vi "Initialize Sessions - 1Sess.vi"(6 "initialize and close session behavior":T2, 7 "visa open timeout":u32, 8 "error in":errorcluster, 9 "access mode":T1 items=["VISA Defaults"=0, "Exclusive Lock"=1, "Load Configured Settings"=4], 10 "instrument type id":string, 11 "session reservation in":refnum<class "Session Reservation.lvclass">) -> (0 "error out":errorcluster, 1 "channel list":string, 2 "session":refnum<visa-resource-name>, 3 "session reservation out":refnum<class "Session Reservation.lvclass">)   [LabVIEW 2020, in "NI Session Management VISA.lvlib"]
doc: "Create a VISA session from the <b>session reservation in</b> and the <b>instrument type id</b>. The <b>instrument type id</b> must match the Instrument Type Id for the custom VISA instrument in the pin map. Returns an error if more than one VISA session has been reserved. Use \"Create Sesssion - NSess.vi\" for multiple sessions."
uses:
  NI Session Management VISA.lvlib
  7f77feb2-d2b5-4acd-8f0f-f1b24b7d1641.vi
  Session Factory/Session Factory.lvclass
  Clients/Session Management V1/Session Reservation/Session Reservation.lvclass
  Clients/Session Management V1/Session Reservation/Initialize and Close Session Behavior.ctl
  <vilib>/Instr/_visa.llb/VISA Open Access Mode.ctl
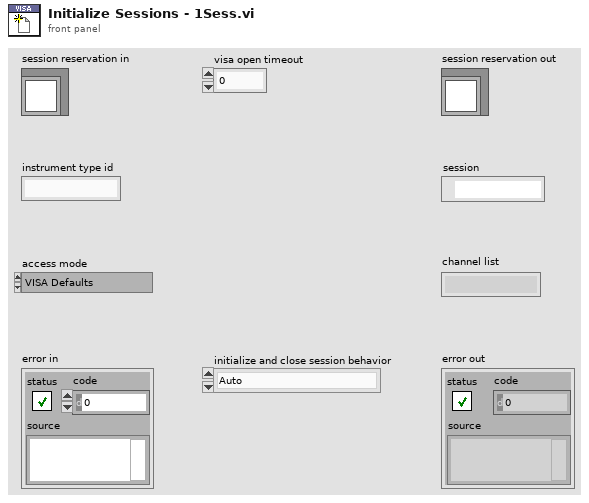
[diagram p1: front panel]
types:
  T1 = typedef "VISA Open Access Mode.ctl" = u32
  T2 = typedef "NI Session Management V1 Client.lvlib/Session Reservation.lvclass/Initialize and Close Session Behavior.ctl" = enum16{"Auto", "Initialize and Close", "Attach and Detach", "Initialize and Detach", "Attach and Close"}
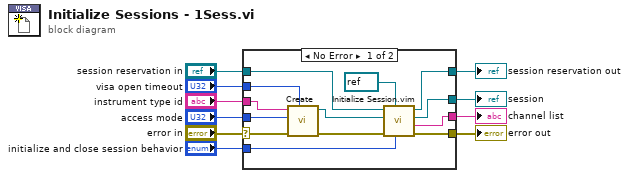
[diagram p0: block diagram]
diagram:
  n1 = case shown="No Error" "error in" {
    selector: "error in" -> [w22 w25]
    tunnel: [w21 w25] -> w9
    tunnel: [w23 w24] -> w7
    tunnel: "session reservation in" -> [w17 w24]
    tunnel: [w20 _] -> w6
    tunnel: [w19 _] -> w4
    tunnel: "initialize and close session behavior" -> [w15 _]
    tunnel: "instrument type id" -> [w13 _]
    tunnel: "access mode" -> [w12 _]
    tunnel: "visa open timeout" -> [w11 _]
    frame No Error {
      n2 = call "Create.vi"("visa open timeout"=w11, "error in"=w22, "access mode"=w12, "instrument type id"=w13) -> ("error out"=w16:errorcluster, "session factory out"=w18:refnum<class "Session Factory.lvclass">)  [unwired: 6 in]
      n3 = call "Initialize Session.vim"("initialize and close session behavior"=w15, "session type"=refnum<visa-resource-name> refnum ("VISA resource name out"), "error in"=w16, "session factory"=w18, "session reservation in"=w17) -> ("error out"=w21:errorcluster, "channel list"=w20:string, "session"=w19:refnum<visa-resource-name>, "session reservation out"=w23:refnum<class "Session Reservation.lvclass">)  [unwired: 3 in]
    }
    frame Error {
    }
  }
  "error out" <- w9
  "session reservation out" <- w7
  "channel list" <- w6
  "session" <- w4
